vi "PH_Interaction.get Systems on same node.vi"(5 "error in":errorcluster) -> (17 "List of systems on the same node":string[](array[string]), 19 "error out":errorcluster)   [LabVIEW 2014, in "PH_Common.lvlib"]
doc: "This VI gets all systems which are running on the same node as the current system."
uses:
  PH_Common.lvlib
  CS_Core/CSSystem/CSSystemLib/CSSystemLib.lvlib
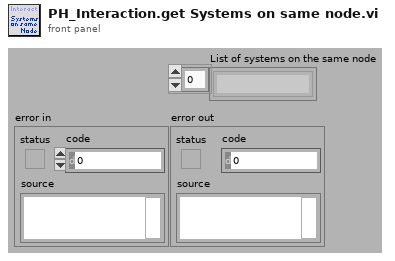
[diagram p1: front panel]
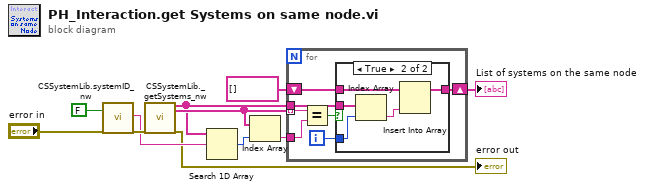
[diagram p0: block diagram]
diagram:
  n1 = call "CSSystemLib.systemID_nw.vi"("set ID"=FALSE, "error in (no error)"="error in") -> ("systemID out"=w8:string, "error out"=w9:errorcluster)  [unwired: 16 in]
  n2 = call "CSSystemLib._getSystems_nw.vi"("error in (no error)"=w9) -> ("CSSystems"=w4:string[], "CSNodes"=w6:string[], "error out"=→"error out":errorcluster)  [unwired: 16 in]
  n3 = Search 1D Array(1D array=w4, element=w8) -> (index of element=w7:i32)  [unwired: 1 in]
  n4 = Index Array(array=w6, index=w7) -> (element=w5:string)
  n5 = for {
    tunnel: w6 -> [w18] mode=indexing
    tunnel: w5 -> [w17]
    tunnel: w4 -> [w16]
    shift-right: [w13] -> w2
    shift-left: string[] [] -> [w12]
    i -> [w14]
    n6 = Equal?(x=w18, y=w17) -> (x = y?=w15:bool)
    n7 = case shown="True" w15 {
      tunnel: w16 -> [_ w24]
      tunnel: w14 -> [_ w23]
      tunnel: [w19 w21] -> w13
      tunnel: w12 -> [w19 w20]
      frame False {
      }
      frame True {
        n8 = Index Array(array=w24, index=w23) -> (element=w22:string)
        n9 = Insert Into Array(array=w20, new element=w22) -> (w21:string[])  [unwired: 1 in]
      }
    }
  }
  "List of systems on the same node" <- w2
